vi "Close Camera.vi"(8 "error in":errorcluster, 10 "Camera Name":string, 11 "Gantry in":refnum<class "Gantry.lvclass">) -> (0 "error out":errorcluster, 3 "Gantry out":refnum<class "Gantry.lvclass">)   [LabVIEW 2017, in "Gantry.lvclass"]
uses:
  Gantry.lvclass
  <vilib>/userdefined/High Color/IMAQdx.ctl
  FlexWorktable/FlexWorktable.lvclass
  <vilib>/vision/driver/NI_Vision_Acquisition_Software.lvlib
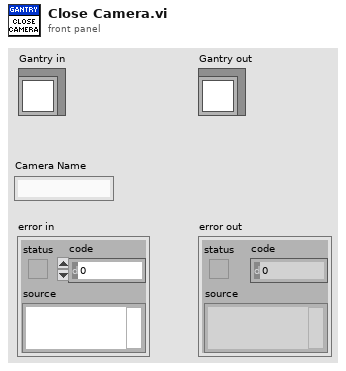
[diagram p1: front panel]
types:
  T1 = typedef "IMAQdx.ctl" = refnum<k21>
  T2 = typedef "FlexWorktable.lvclass/Camera State.ctl" = cluster{"Group":i32, "Open?":bool, "Interface Name":string, "Field of View":cluster{"x-mm":dbl, "y-mm":dbl}}
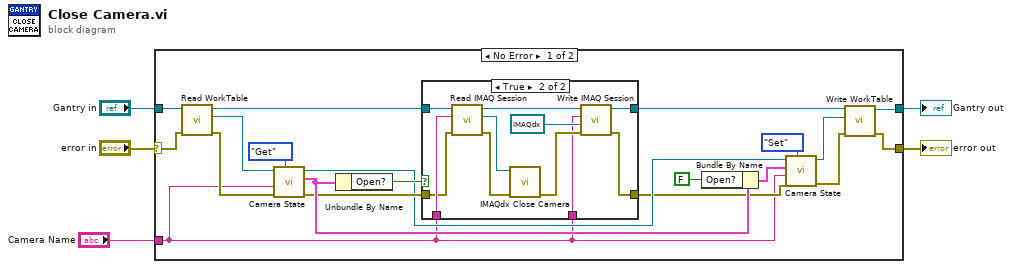
[diagram p0: block diagram]
diagram:
  n1 = case shown="No Error" "error in" {
    selector: "error in" -> [w21 w40]
    tunnel: [w9 w40] -> w4
    tunnel: [w8 w39] -> w2
    tunnel: "Gantry in" -> [w25 w39]
    tunnel: "Camera Name" -> [w6 _]
    frame No Error {
      n2 = call-dynamic "Read WorkTable.vi"("error in"=w21, "Gantry Class in"=w25) -> ("error out"=w20:errorcluster, "Worktable"=w24:refnum<class "FlexWorktable.lvclass">, "Gantry Class out"=w19:refnum<class "Gantry.lvclass">)  [unwired: 7 in]
      n3 = call-dynamic "Camera State.vi"("Get/Set"=enum16{"Get", "Set"}."Get", "error in (no error)"=w20, "Camera Name"=w6, "FlexWorktable in"=w24) -> ("error out"=w16:errorcluster, "State"=w23:T2, "FlexWorktable out"=w15:refnum<class "FlexWorktable.lvclass">)  [unwired: 5 in]
      n4 = Unbundle By Name(w23) -> ("Open?"=w17:bool)
      n5 = case shown="True" w17 {
        tunnel: w19 -> [w26 w38]
        tunnel: w6 -> [_ w36]
        tunnel: w16 -> [w27 w33]
        tunnel: [w27 w30] -> w13
        tunnel: [w26 w29] -> w12
        tunnel: w6 -> [_ w28]
        frame False {
        }
        frame True {
          n6 = call-dynamic "Read IMAQ Session.vi"("error in (no error)"=w33, "Camera Name"=w36, "Gantry Class in"=w38) -> ("error out"=w32:errorcluster, "IMAQ Session"=w37:T1, "Gantry Class out"=w34:refnum<class "Gantry.lvclass">)  [unwired: 6 in]
          n7 = call <vilib>:"IMAQdx Close Camera.vi"("error in"=w32, "Session In"=w37) -> ("error out"=w31:errorcluster)  [unwired: 9 in]
          n8 = call-dynamic "Write IMAQ Session.vi"("error in (no error)"=w31, "IMAQ Session"=T1 refnum, "Camera Name"=w28, "Gantry Class in"=w34) -> ("error out"=w30:errorcluster, "Gantry Class out"=w29:refnum<class "Gantry.lvclass">)  [unwired: 6 in]
        }
      }
      n9 = Bundle By Name(cluster=w23, "Open?"=FALSE) -> (w14:T2)
      n10 = call-dynamic "Camera State.vi"("Get/Set"=enum16{"Get", "Set"}."Set", "error in (no error)"=w13, "Camera Name"=w6, "New State"=w14, "FlexWorktable in"=w15) -> ("error out"=w10:errorcluster, "FlexWorktable out"=w11:refnum<class "FlexWorktable.lvclass">)  [unwired: 4 in, 1 out]
      n11 = call-dynamic "Write WorkTable.vi"("error in (no error)"=w10, "FlexWorktable"=w11, "Gantry Class in"=w12) -> ("error out"=w9:errorcluster, "Gantry Class out"=w8:refnum<class "Gantry.lvclass">)  [unwired: 7 in]
    }
    frame Error {
    }
  }
  "error out" <- w4
  "Gantry out" <- w2
